vi "GetPos.vi"(6 "Position 2":refnum<vi>, 8 "error in (no error)":errorcluster, 11 "QuickSilver in":refnum<class "QuickSilver.lvclass">) -> (0 "error out":errorcluster, 2 "Position":dbl, 3 "QuickSilver out":refnum<class "QuickSilver.lvclass">)   [LabVIEW 2012, in "QuickSilver.lvclass"]
uses:
  QuickSilver.lvclass
  QuickSilver.lvclass/QuickSilver.ctl
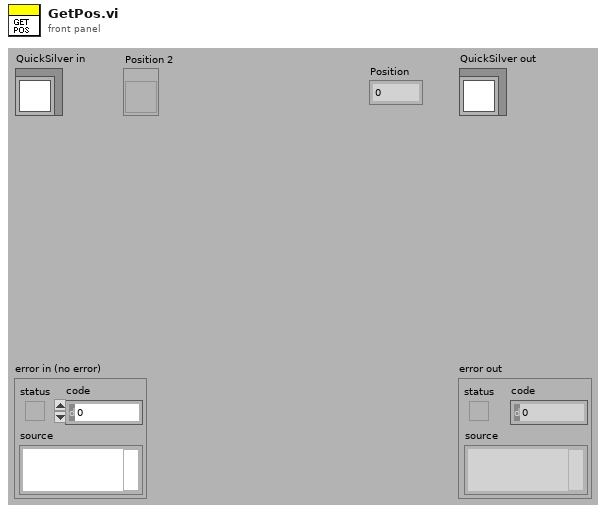
[diagram p1: front panel]
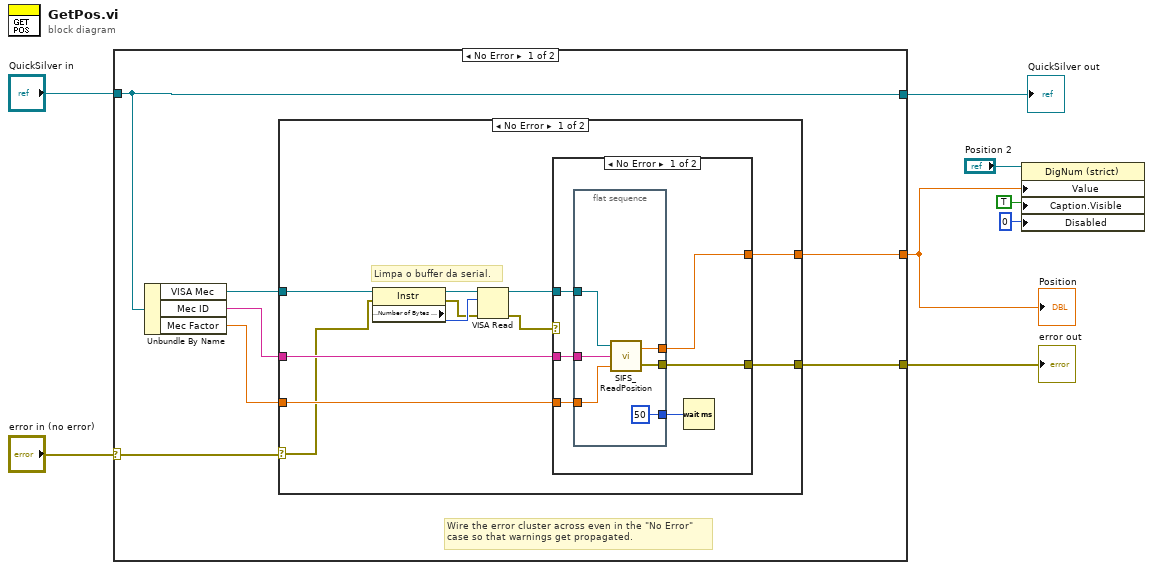
[diagram p0: block diagram]
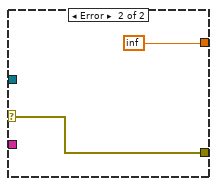
[diagram p2: hidden frame]
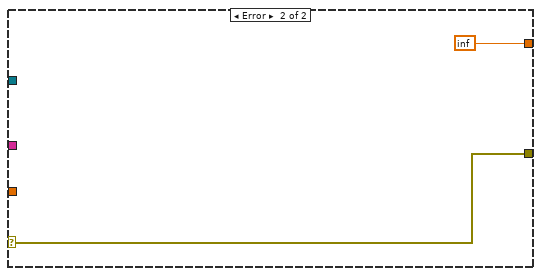
[diagram p3: hidden frame]
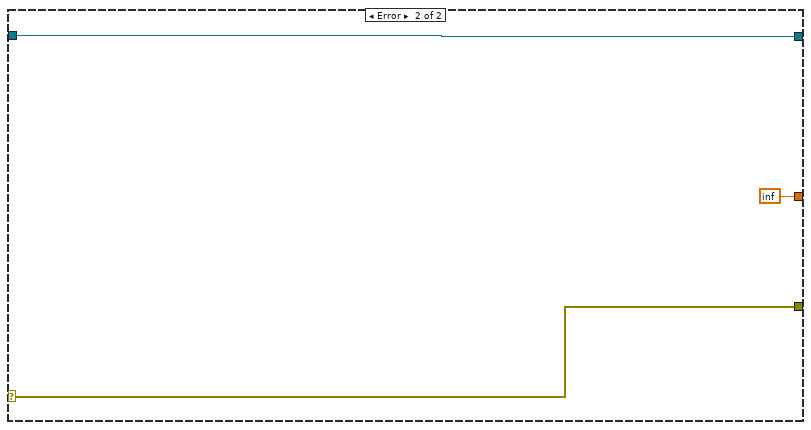
[diagram p4: hidden frame]
diagram:
  n1 = case shown="No Error" "error in (no error)" {
    selector: "error in (no error)" -> [w13 w45]
    tunnel: [w15 w45] -> w7
    tunnel: [w12 w44] -> w6
    tunnel: "QuickSilver in" -> [w12 w44]
    tunnel: [w14 inf] -> w4
    frame No Error {
      # "Wire the error cluster across even in the \"No Error\"\ncase so that warnings get propagated."
      n2 = Unbundle By Name(w12) -> ("VISA Mec"=w11:refnum<visa-resource-name>, "Mec ID"=w10:string, "Mec Factor"=w9:dbl)
      n3 = case shown="No Error" w13 {
        selector: w13 -> [w21 w42]
        tunnel: [w25 w42] -> w15
        tunnel: [w24 inf] -> w14
        tunnel: w9 -> [w23 _]
        tunnel: w11 -> [w19 _]
        tunnel: w10 -> [w22 _]
        frame No Error {
          # "Limpa o buffer da serial."
          n4 = property class="Instr"(reference=w19, error in=w21) -> (reference out=w18:refnum<visa-resource-name>, error out=w16:errorcluster, "Serial Settings:Number of Bytes at Serial Port"=w17:u32)
          n5 = VISA Read(VISA resource name=w18, byte count=w17, error in (no error)=w16) -> (VISA resource name out=w26:refnum<visa-resource-name>, error out=w20:errorcluster)  [unwired: 2 out]
          n6 = case shown="No Error" w20 {
            selector: w20 -> [_ w40]
            tunnel: w26 -> [w32 _]
            tunnel: [w31 w40] -> w25
            tunnel: [w30 inf] -> w24
            tunnel: w23 -> [w29 _]
            tunnel: w22 -> [w28 _]
            frame No Error {
              n7 = flat-sequence {
                tunnel: w32 -> [w38]
                tunnel: w29 -> [w37]
                tunnel: w28 -> [w34]
                tunnel: [u32 50 ("milliseconds to wait")] -> w27
                tunnel: [w36] -> w30
                tunnel: [w35] -> w31
                frame #0 {
                  n8 = call "SIFS_ReadPosition.vi"("FATOR"=w37, "ID"=w34, "VISA resource name"=w38) -> ("error out"=w35:errorcluster, "Position"=w36:dbl)
                }
              }
              n9 = Wait (ms)(milliseconds to wait=w27) -> ()  [unwired: 1 out]
            }
            frame Error {
            }
          }
        }
        frame Error {
        }
      }
    }
    frame Error {
    }
  }
  "error out" <- w7
  "QuickSilver out" <- w6
  "Position" <- w4
  n10 = property class="DigNum (strict)"(reference="Position 2", "Value"=w4, "Caption.Visible"=TRUE, "Disabled"=u8 0) -> ()  [unwired: 1 in, 2 out]
